vi "GetRxPower-Debug.vi"(0 "SAVE FILE PATH":path, 1 "SHOW PLOT(T)":bool, 5 "CloseCOM4":bool=TRUE, 7 "RunAM_Init":bool, 9 "UseFastData(T)":bool, 11 "error in (no error)":errorcluster, 12 "SAVE TO FILE(T)":bool, 13 "CF(MHZ)":dbl=10.0 min=0.0 max=150.0 format="%#_13g", 14 "BW(MHZ)":dbl=10.0 format="%#_13g") -> (2 "band (dbfs/mhz)":dbl[](array[numeric])=[-46.7, 9.965], 3 "peak (dbfs/mhz)":dbl[](array[numeric])=[-17.4, 19.85], 15 "error out":errorcluster)   [LabVIEW 2018]
panel:
  out "x+1":i32
  out "peak (dbfs/mhz) 2":dbl[](array[numeric])=[-17.4, 19.85]
  in  "stop":bool
  in  "Numeric":i32
  out "Array":dbl[][](array[numeric])
  out "standard output":string
  out "Time(ms)":u32
  out "start":u32
  in  "INPUT FROM FILE(T)":bool
  in  "INPUT FILE PATH":path
  out "console  output":string="Max Value: -17.492 dBFS at 19.858 MHz\r\nCF_OUT(MHz) = 9.96580361504641\r\nBP_OUT(dBfs) = -46.72236447882276\r\n"
  # "Input Dialog. Check \"Show Plot\" if desired"
  # "File Path Dialog. Check if file save desired"
  # "Band  & Peak Power Outputs"
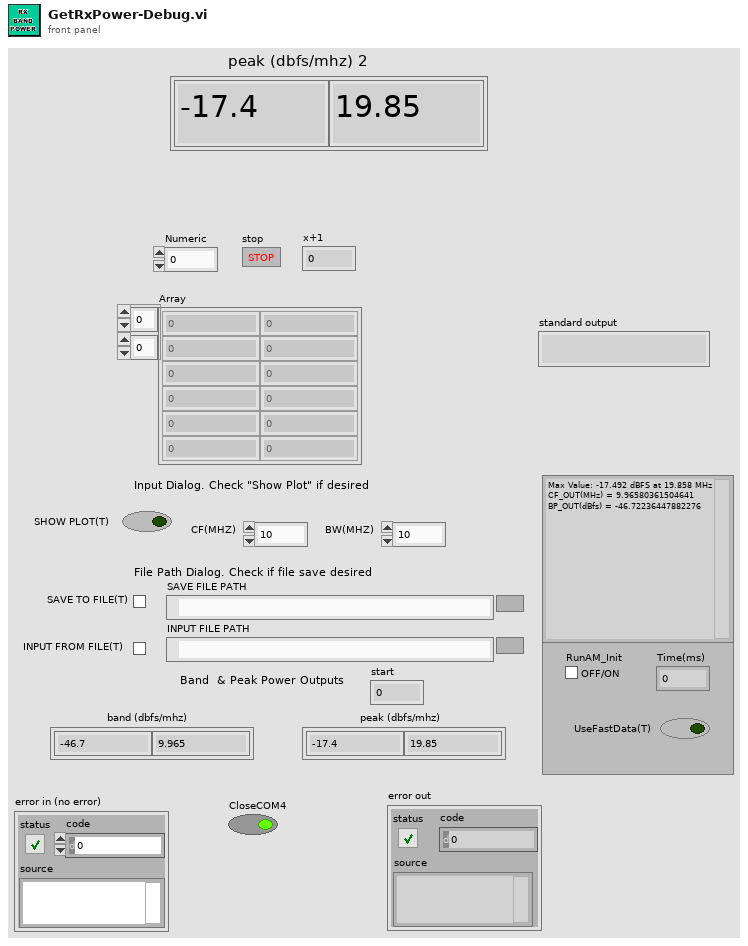
[diagram p1: front panel]
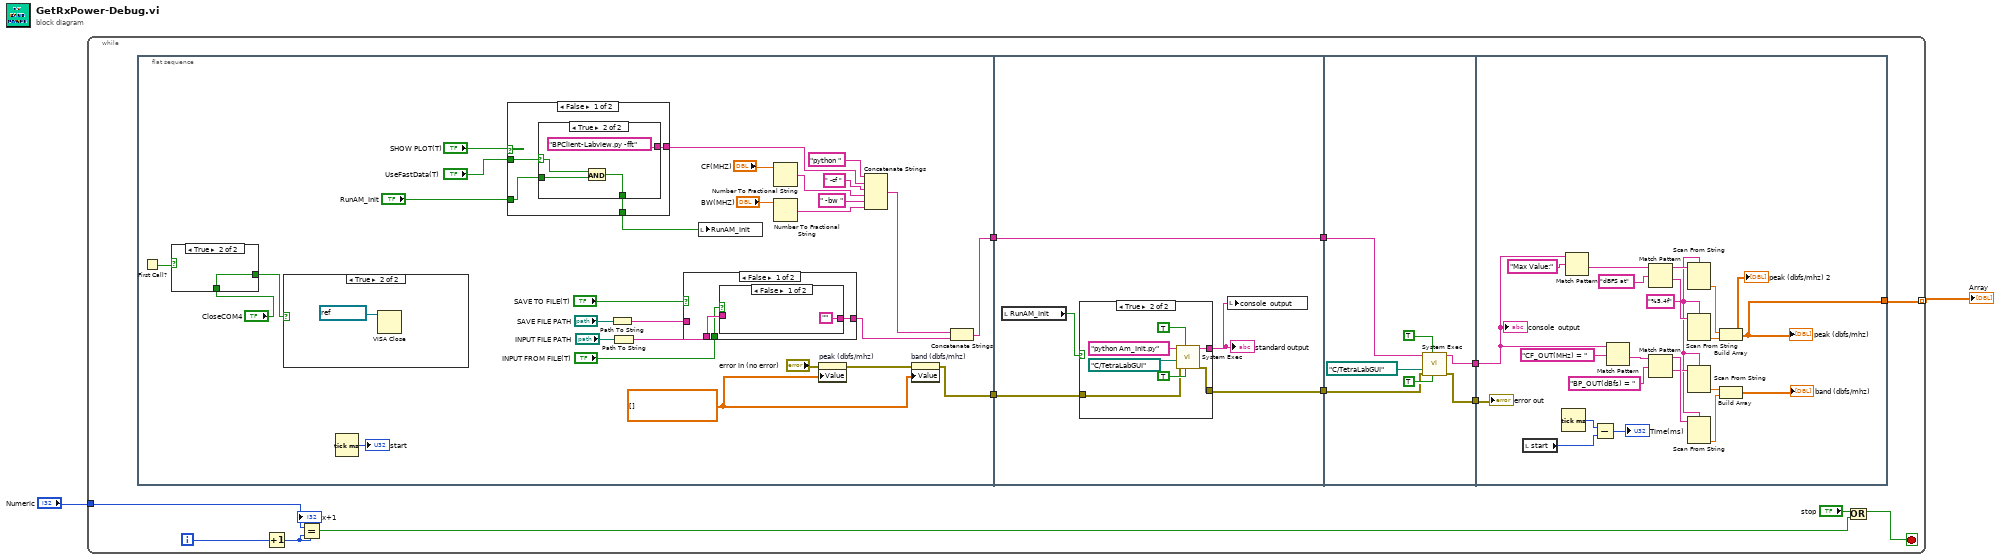
[diagram p0: block diagram]
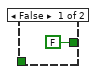
[diagram p2: hidden frame]
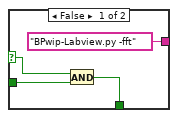
[diagram p4: hidden frame]
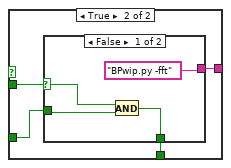
[diagram p5: hidden frame]
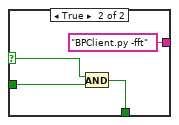
[diagram p6: hidden frame]
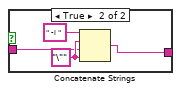
[diagram p7: hidden frame]
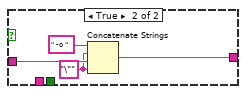
[diagram p8: hidden frame]
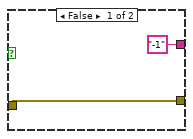
[diagram p9: hidden frame]
diagram:
  n1 = while {
    tunnel: [w9] -> w2 mode=indexing
    tunnel: "Numeric" -> [w5]
    i -> [w6]
    stop <- w7 stop-if-true
    n2 = flat-sequence {
      tunnel: [w23] -> w15
      tunnel: [w24] -> w14
      tunnel: [w88] -> w13
      tunnel: [w87] -> w12
      tunnel: w15 -> [w88]
      tunnel: w14 -> [w86]
      tunnel: [w100] -> w11
      tunnel: [w99] -> w10
      tunnel: w13 -> [w101]
      tunnel: w12 -> [w98]
      tunnel: w11 -> [w124]
      tunnel: w10 -> [w109]
      tunnel: [w105] -> w9
      frame #0 {
        w28 = dbl[] [] ("peak (dbfs/mhz)")
        n3 = First Call?() -> (First Call?: T/F=w16:bool)
        n4 = case shown="True" w16 {
          tunnel: "CloseCOM4" -> [_ w46]
          tunnel: [FALSE ("CloseCOM4") w46] -> w17
          frame False {
          }
          frame True {
          }
        }
        n5 = case shown="True" w17 {
          frame False {
          }
          frame True {
            n6 = VISA Close(VISA resource name=refnum<visa-resource-name> "COM4") -> ()  [unwired: 1 in, 1 out]
          }
        }
        n7 = Tick Count (ms)() -> (millisecond timer value=→"start":u32)
        n8 = case shown="False" "SHOW PLOT(T)" {
          tunnel: [w51 w63] -> w33
          tunnel: "UseFastData(T)" -> [w48 w62]
          tunnel: [w50 w61] -> w21
          tunnel: "RunAM_Init" -> [w49 w60]
          frame False {
            n9 = case shown="True" w48 {
              selector: w48 -> [w52 w56]
              tunnel: ["BPwip-Labview.py -fft" ("command line") "BPClient-Labview.py -fft" ("command line")] -> w51
              tunnel: [w54 w57] -> w50
              tunnel: w49 -> [w53 w58]
              frame False {
                n10 = And(x=w52, y=w53) -> (x .and. y?=w54:bool)
              }
              frame True {
                n11 = And(x=w56, y=w58) -> (x .and. y?=w57:bool)
              }
            }
          }
          frame True {
            n12 = case shown="False" w62 {
              selector: w62 -> [w65 w69]
              tunnel: ["BPwip.py -fft" ("command line") "BPClient.py -fft" ("command line")] -> w63
              tunnel: [w66 w70] -> w61
              tunnel: w60 -> [w64 w68]
              frame False {
                n13 = And(x=w65, y=w64) -> (x .and. y?=w66:bool)
              }
              frame True {
                n14 = And(x=w69, y=w68) -> (x .and. y?=w70:bool)
              }
            }
          }
        }
        n15 = Path To String(path="SAVE FILE PATH") -> (string=w29:string)
        n16 = Path To String(path="INPUT FILE PATH") -> (string=w43:string)
        n17 = case shown="False" "SAVE TO FILE(T)" {
          tunnel: w29 -> [_ w83]
          tunnel: [w74 w82] -> w38
          tunnel: w43 -> [w73 _]
          tunnel: "INPUT FROM FILE(T)" -> [w72 _]
          frame False {
            n18 = case shown="False" w72 {
              tunnel: ["" w77] -> w74
              tunnel: w73 -> [_ w76]
              frame False {
              }
              frame True {
                w78 = "\"" ("string")
                n19 = Concatenate Strings(" -i " ("string"), w78, w76, w78) -> (w77:string)
              }
            }
          }
          frame True {
            w80 = "\"" ("string")
            n20 = Concatenate Strings(" -o " ("string"), w80, w83, w80) -> (w82:string)
          }
        }
        n21 = local write "RunAM_Init"(w21) -> ()
        n22 = Number To Fractional String(number="CF(MHZ)") -> (F-format string=w34:string)  [unwired: 3 in]
        n23 = Number To Fractional String(number="BW(MHZ)") -> (F-format string=w35:string)  [unwired: 3 in]
        n24 = property on="peak (dbfs/mhz)" class="Arr (strict)"(error in="error in (no error)", "Value"=w28) -> (error out=w41:errorcluster)  [unwired: 1 in, 1 out]
        n25 = Concatenate Strings("python " ("string"), w33, " -cf " ("string"), w34, " -bw " ("string"), w35) -> (w36:string)
        n26 = property on="band (dbfs/mhz)" class="Arr (strict)"(error in=w41, "Value"=w28) -> (error out=w24:errorcluster)  [unwired: 1 in, 1 out]
        n27 = Concatenate Strings(w36, w38) -> (w23:string)
      }
      frame #1 {
        n28 = local read "RunAM_Init"() -> (w85:bool)
        n29 = case shown="True" w85 {
          tunnel: [w90 w95] -> w87
          tunnel: w86 -> [w90 w92]
          tunnel: ["-1" ("standard output") w91] -> w84
          frame False {
          }
          frame True {
            n30 = call <vilib>:"System Exec.vi"("run minimized? (F)"=TRUE, "wait until completion? (T)"=TRUE, "error in (no error)"=w92, "working directory"=path "C:/TetraLabGUI", "command line"="python Am_Init.py") -> ("error out"=w95:errorcluster, "standard output"=w91:string)  [unwired: 3 in, 2 out]
          }
        }
        "standard output" <- w84
        n31 = local write "console  output"(w84) -> ()
      }
      frame #2 {
        n32 = call <vilib>:"System Exec.vi"("run minimized? (F)"=TRUE, "wait until completion? (T)"=TRUE, "error in (no error)"=w98, "working directory"=path "C:/TetraLabGUI", "command line"=w101) -> ("error out"=w99:errorcluster, "standard output"=w100:string)  [unwired: 3 in, 2 out]
      }
      frame #3 {
        w113 = "%5.4f" ("format string")
        n33 = local read "start"() -> (w107:u32)
        n34 = Tick Count (ms)() -> (millisecond timer value=w108:u32)
        n35 = Match Pattern(string=w124, regular expression="Max Value:") -> (after substring=w120:string)  [unwired: 1 in, 3 out]
        n36 = Subtract(x=w108, y=w107) -> (x-y=→"Time(ms)":u32)
        n37 = Match Pattern(string=w124, regular expression="CF_OUT(MHz) = ") -> (after substring=w116:string)  [unwired: 1 in, 3 out]
        n38 = Match Pattern(string=w120, regular expression="dBFS at") -> (before substring=w121:string, after substring=w122:string)  [unwired: 1 in, 2 out]
        n39 = Match Pattern(string=w116, regular expression="BP_OUT(dBfs) = ") -> (before substring=w115:string, after substring=w114:string)  [unwired: 1 in, 2 out]
        n40 = Scan From String(format string=w113, input string=w121) -> (output 1=w125:dbl)  [unwired: 3 in, 3 out]
        n41 = Scan From String(format string=w113, input string=w122) -> (output 1=w126:dbl)  [unwired: 3 in, 3 out]
        n42 = Scan From String(format string=w113, input string=w114) -> (output 1=w111:dbl)  [unwired: 3 in, 3 out]
        n43 = Scan From String(format string=w113, input string=w115) -> (output 1=w110:dbl)  [unwired: 3 in, 3 out]
        n44 = Build Array(w125, w126) -> (w105:dbl[])
        "peak (dbfs/mhz)" <- w105
        "peak (dbfs/mhz) 2" <- w105
        n45 = Build Array(w111, w110) -> (→"band (dbfs/mhz)":dbl[])
        "console  output" <- w124
        "error out" <- w109
      }
    }
    n46 = Increment(x=w6) -> (x+1=w4:i32)
    "x+1" <- w4
    n47 = Equal?(x=w5, y=w4) -> (x = y?=w3:bool)
    n48 = Or(x="stop", y=w3) -> (x .or. y?=w7:bool)
  }
  "Array" <- w2
